vi "Handler Launch Failure.vi"(8 "error in (no error)":errorcluster) -> (0 "error out":errorcluster)   [LabVIEW 2021, in "TCP Slave.lvclass"]
doc: "Displays a message which lets the user know that an error has occured when launching the slave."
uses:
  TCP Slave.lvclass
  TCP Slave.lvclass/TCP Slave.ctl
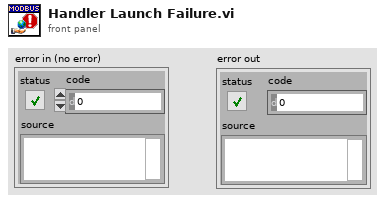
[diagram p1: front panel]
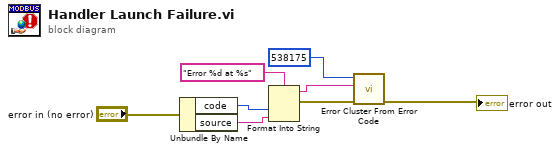
[diagram p0: block diagram]
diagram:
  n1 = Unbundle By Name("error in (no error)") -> ("code"=w5:i32, "source"=w6:string)
  n2 = Format Into String(format string="Error %d at %s", w5, w6) -> (resulting string=w3:string, error out=w7:errorcluster)  [unwired: 2 in]
  n3 = call <vilib>:"Error Cluster From Error Code.vi"("error in (no error)"=w7, "error message (\"\")"=w3, "error code (0)"=538175) -> ("error out"=→"error out":errorcluster)  [unwired: 6 in]
